vi "GEOM_GeomMngr.vi"(5 "calc headers?":bool=TRUE, 6 "arguments":string[](array[string]), 7 "hdrmodspath":path=path "kk", 8 "error in (no error)":errorcluster, 9 "switches":string[](array[string]), 10 "command":string, 11 "database path":path=path "/home/ArcVIEW/Modules/GEOM/public/database") -> (0 "error out":errorcluster, 2 "response":string)   [LabVIEW 2016]
uses:
  GEOM_Coords.ctl
  GEOM_FPAReadMode.ctl
  GEOM_Amplifier.ctl
  GEOM_AmpType.ctl
  GEOM_ROI.ctl
  GEOM_ROICorrection.ctl
  GEOM_CoordsRef.ctl
  GEOM_VAR_action.ctl
  GEOM_Gbls.vi
panel:
  out "ref":T1
  in  "GEOM_coordsref":T1
  out "lastformat":string
  in  "BinCorrectionType":T2(ring)
  out "last readmode":string
  in  "CorrectionType":T3
  in  "FPAReadMode":T4 {"Amplifiers"."fliped" items=["none", "horizontal", "vertical"]; "Amplifiers"."type" items=["LL", "LR", "UL", "UR"]}
  in  "ROIcoords":T8={"xstart"=1, "ystart"=1, "xsize"=1, "ysize"=1}
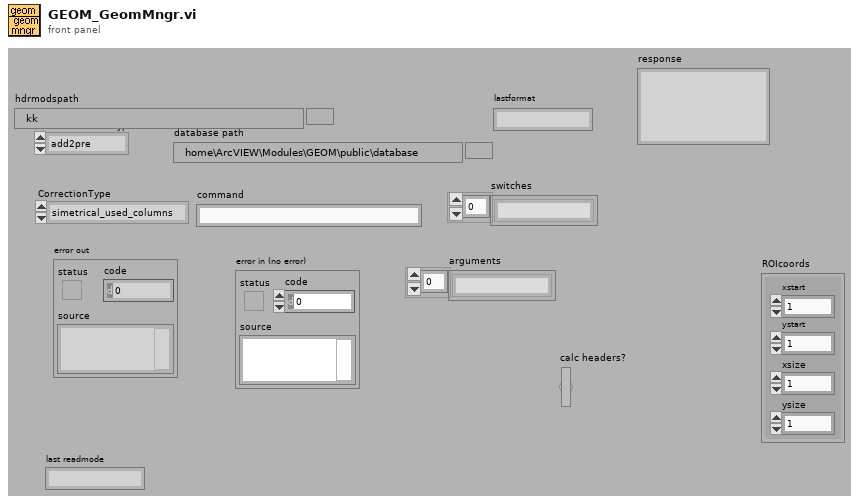
[diagram p1: front panel]
types:
  T1 = typedef "GEOM_CoordsRef.ctl" = cluster{"xref":u32, "yref":u32}
  T2 = enum16{"add2pre", "add2post", "add2data", "none"}
  T3 = typedef "GEOM_ROICorrection.ctl" = enum16{"simetrical_used_columns", "simetrical_all_columns"}
  T4 = typedef "GEOM_FPAReadMode.ctl" = cluster{"name":string, "Amplifiers":T5[]}
  T5 = typedef "GEOM_Amplifier.ctl" = cluster{"number":i32, "type":T6, "rotated":i16, "fliped":u16, "FPAcoord":cluster{"xstart":i32, "ystart":i32}, "Physical_size":cluster{"columns":i32, "rows":i32}, "predata":cluster{"columns":i32, "rows":i32}, "postdata":cluster{"columns":i32, "rows":i32}, "Req ROIs":T7, "Corr ROI":T7, "Detnumber":i32, "ampID":string, "discard":i32}
  T6 = typedef "GEOM_AmpType.ctl" = u16
  T7 = typedef "GEOM_ROI.ctl" = T8[]
  T8 = typedef "GEOM_Coords.ctl" = cluster{"xstart":u32, "ystart":u32, "xsize":u32, "ysize":u32}
  T9 = typedef "GEOM_VAR_action.ctl" = enum16{"read", "write"}
  T10 = typedef "DatabaseHand_RefNum.ctl" = refnum<vi>
  T11 = typedef "GEOM_AmpModifiers.ctl" = cluster{"Binning":T12, "sections":T13[]}
  T12 = typedef "GEOM_Binning.ctl" = cluster{"x":u32, "y":u32}
  T13 = typedef "GEOM_Moifier.ctl" = cluster{"name":string, "header section":string, "comment":string, "value":i32, "binning?":bool, "Where":enum16{"predata", "postdata"}, "add In":enum16{"columns", "rows", "none"}}
  T14 = typedef "GEOM_FPADetectors.ctl" = T15[]
  T15 = typedef "GEOM_DetStruct.ctl" = cluster{"name":string, "number":i32, "Info":string[][], "ReadModes":T16[], "detxpos":i32, "detypos":i32, "detcols":i32, "detrows":i32, "discard":i32}
  T16 = typedef "GEOM_ReadMode.ctl" = cluster{"name":string, "amplifiers":T5[], "nxamps":i32, "nyamps":i32}
  T17 = cluster{"FPA":string, "Info":string[][], "Sorted Detectors":T14}
  T18 = typedef "GEOM_DetSummaryStruct.ctl" = cluster{"detxpos":i32, "detypos":i32, "cols":i32, "rows":i32, "nxamps":i32, "nyamps":i32, "number":i32, "discard":i32, "totcols":i32, "totrows":i32, "readmode":string}
  T19 = typedef "GEOM_CorrectedFPA.ctl" = cluster{"readmode":string, "amplifiers":cluster{"number":i32, "xstart":i32, "ystart":i32}[], "totxsize":i32, "totysize":i32, "maxxdim":i32, "maxydim":i32, "numxamps":i32, "numyamps":i32, "totxdata":i32, "totydata":i32, "xdataamp":i32, "ydataamp":i32, "totpixels":i32}
  T20 = cluster{"name":string, "header section":string, "comment":string, "value":i32, "binning?":bool, "Where":enum16{"predata", "postdata"}, "add In":enum16{"columns", "rows", "none"}}[]
  T21 = cluster{"Amplifiers":T5[], "BinFPA":T19, "detreadmode":cluster{"name":string, "detectors":T18[]}}
  T22 = typedef "GEOM_HeaderModule.ctl" = cluster{"name":string, "Keys":string[][]}
  T23 = typedef "GEOM_HdrSec.ctl" = cluster{"name":string, "directives":T24, "comment":string, "amptype":enum16{"LL", "LR", "UL", "UR", "ALL", "LEFT", "RIGHT", "UPPER", "LOWER"}, "ampid":bool, "detid":bool, "unbin":bool}
  T24 = typedef "GEOM_CoorSys.ctl" = cluster{"coords":string, "reference":string, "xarea":string, "yarea":string, "order":string}
  T25 = typedef "GEOM_FormatGeomkeys.ctl" = cluster{"inienclose":string, "endenclose":string, "rangesep":string, "secsep":string}
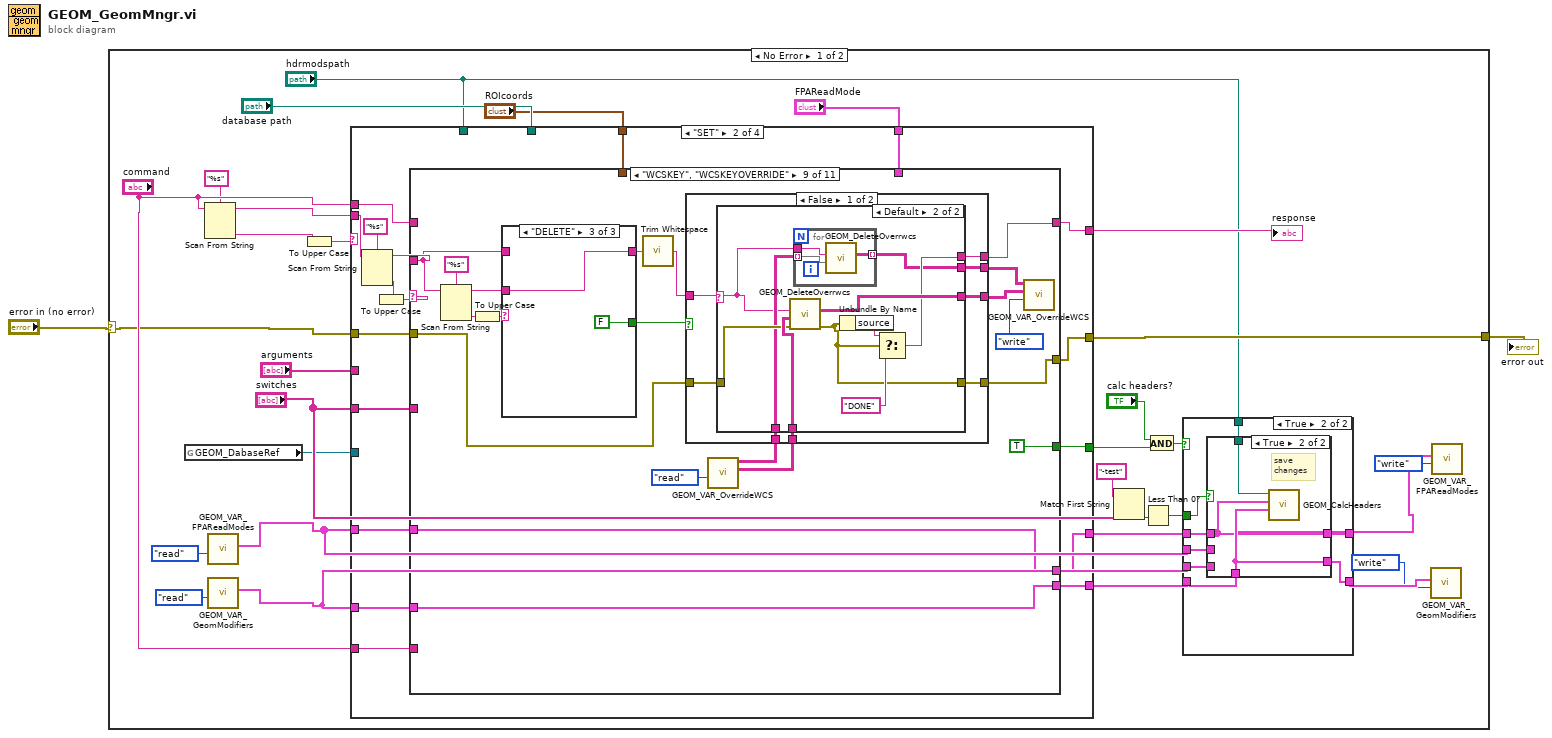
[diagram p0: block diagram]
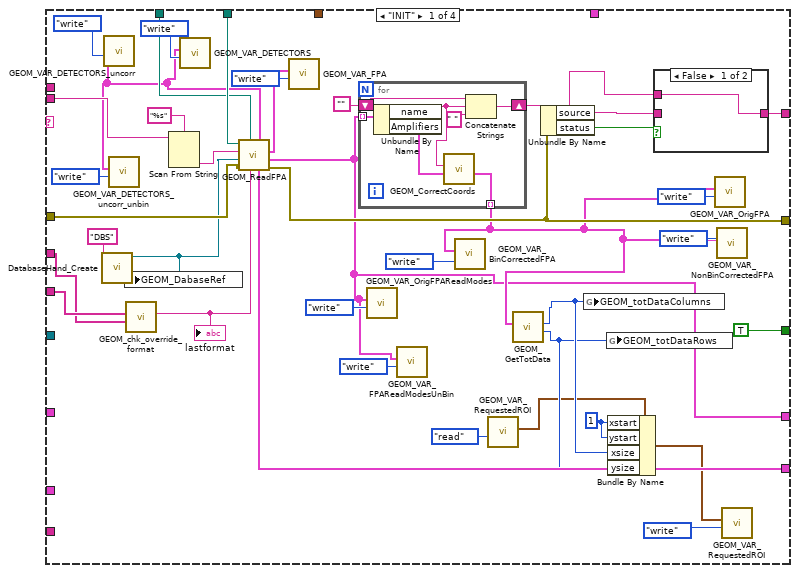
[diagram p2: hidden frame]
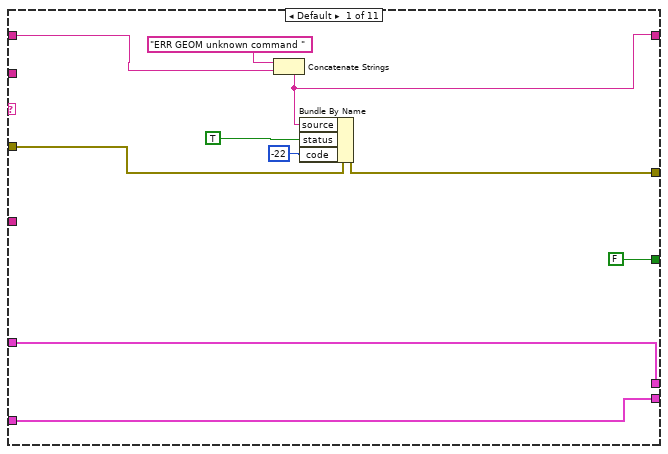
[diagram p4: hidden frame]
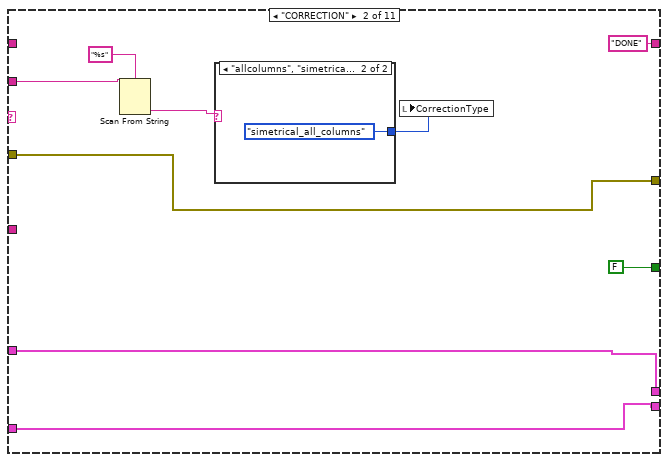
[diagram p5: hidden frame]
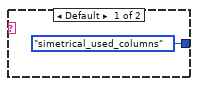
[diagram p6: hidden frame]
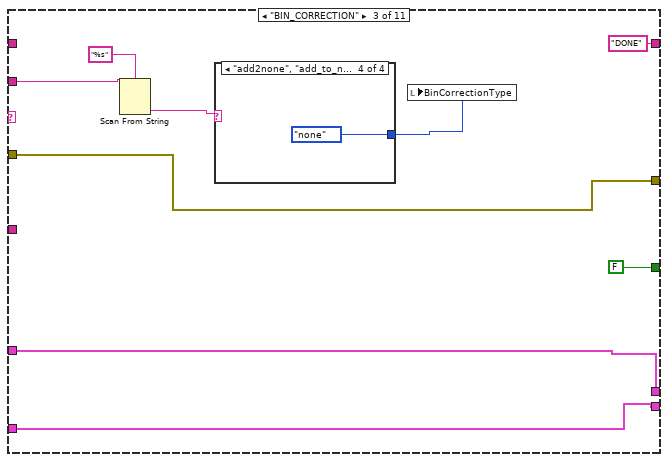
[diagram p7: hidden frame]
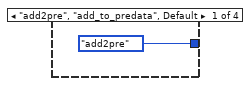
[diagram p8: hidden frame]
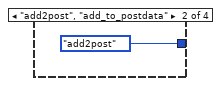
[diagram p9: hidden frame]
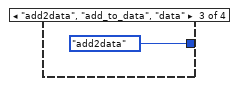
[diagram p10: hidden frame]
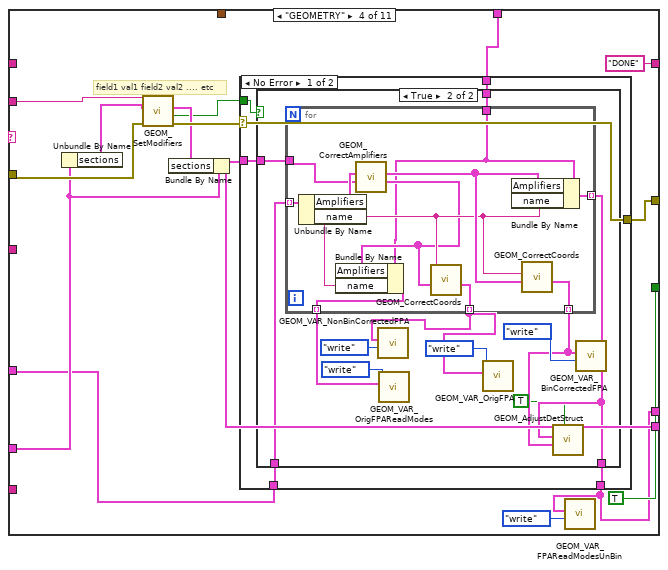
[diagram p11: hidden frame]
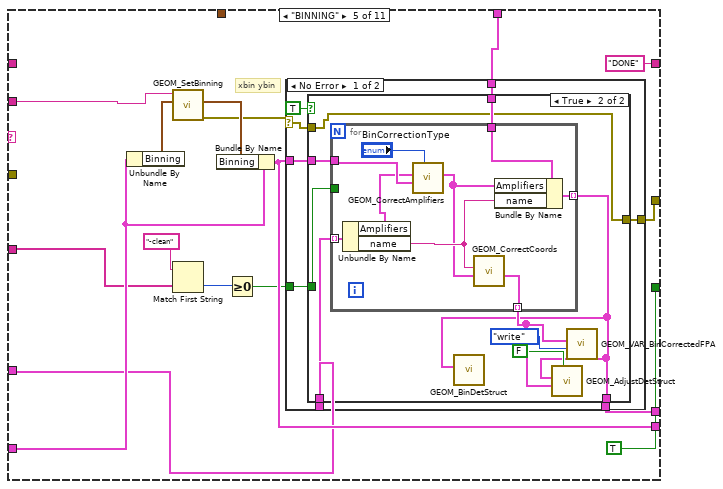
[diagram p14: hidden frame]
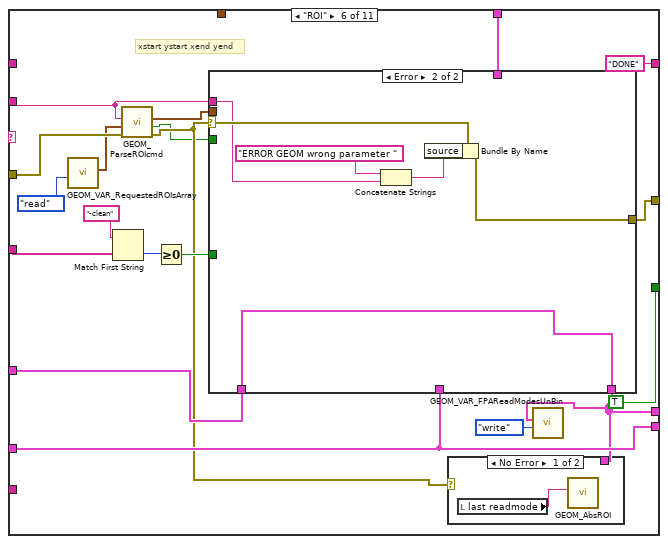
[diagram p17: hidden frame]
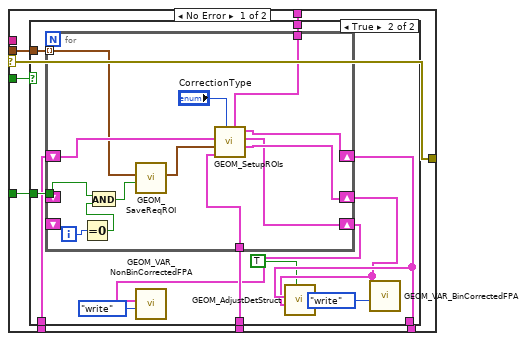
[diagram p19: hidden frame]
diagram:
  n1 = case shown="No Error" "error in (no error)" {
    selector: "error in (no error)" -> [w19 w727]
    tunnel: [w20 w727] -> w2
    frame No Error {
      n2 = global read "GEOM_Gbls.vi" "GEOM_DabaseRef"() -> (w18:T10)
      n3 = Scan From String(format string="%s", input string="command") -> (remaining string=w25:string, output 1=w26:string)  [unwired: 2 in, 3 out]
      n4 = call "GEOM_VAR_FPAReadModes.vi"("Action"=GEOM_VAR_action."read") -> ("GEOM_FPAReadModes out"=w14:T4[])  [unwired: 1 in, 9 out]
      n5 = call "GEOM_VAR_GeomModifiers.vi"("Action"=GEOM_VAR_action."read") -> ("GEOM_modifiers out"=w10:T11)  [unwired: 1 in, 9 out]
      n6 = To Upper Case(1:w26) -> (0:w7:string)
      n7 = case shown="\"SET\"" w7 {
        tunnel: "database path" -> [w72 _ _ _]
        tunnel: w19 -> [w39 w97 w409 w709]
        tunnel: [w67 w96 w408 w708] -> w20
        tunnel: w25 -> [w69 w95 w406 _]
        tunnel: "command" -> [_ w94 _ w706]
        tunnel: "switches" -> [w56 w86 _ _]
        tunnel: "ROIcoords" -> [_ w92 _ _]
        tunnel: "FPAReadMode" -> [_ w91 _ _]
        tunnel: w14 -> [_ w90 w410 w710]
        tunnel: [w34 w89 w410 w710] -> w22
        tunnel: w10 -> [_ w88 w407 w707]
        tunnel: [w68 w87 w407 w707] -> w21
        tunnel: [w65 w85 w411 w711] -> w29
        tunnel: "command" -> [_ w84 _ _]
        tunnel: w18 -> [_ _ w404 _]
        tunnel: "arguments" -> [w55 _ _ _]
        tunnel: "hdrmodspath" -> [w44 _ w400 _]
        tunnel: [TRUE ("x") w82 w401 FALSE ("x")] -> w6
        frame "INIT" {
          w60 = u32 1 ("xstart")
          n8 = call "DatabaseHand_Create.vi"("Name"="DBS") -> ("Database RefNum out"=w38:T10)  [unwired: 1 in, 9 out]
          n9 = global write "GEOM_Gbls.vi" "GEOM_DabaseRef"(w38) -> ()
          n10 = call "GEOM_chk_override_format.vi"("arguments"=w55, "switches"=w56) -> ("format out"=w57:string)  [unwired: 9 out]
          "lastformat" <- w57
          n11 = Scan From String(format string="%s", input string=w69) -> (output 1=w70:string)  [unwired: 2 in, 4 out]
          n12 = call "GEOM_ReadFPA.vi"("override format"=w57, "moddir"=w44, "error in (no error)"=w39, "Database RefNum out"=w38, "FPA"=w70, "database path"=w72) -> ("error out"=w67:errorcluster, "FPAReadModes"=w34:T4[], "FPA"=w49:T17, "modifiers"=w68:T11, "detreadmodes"=w36:cluster{"name":string, "detectors":T18[]}[])  [unwired: 1 out]
          n13 = call "GEOM_VAR_DETECTORS_uncorr.vi"("Action"=GEOM_VAR_action."write", "det in"=w36) -> ()  [unwired: 10 out]
          n14 = call "GEOM_VAR_DETECTORS_uncorr_unbin.vi"("Action"=GEOM_VAR_action."write", "det in"=w36) -> ()  [unwired: 10 out]
          n15 = call "GEOM_VAR_DETECTORS.vi"("Action"=GEOM_VAR_action."write", "det in"=w36) -> ()  [unwired: 10 out]
          n16 = call "GEOM_VAR_FPA.vi"("Action"=GEOM_VAR_action."write", "GEOM_FPA"=w49) -> ()  [unwired: 10 out]
          n17 = for {
            tunnel: w34 -> [w79] mode=indexing
            shift-right: [w77] -> w62
            shift-left: "" -> [w78]
            tunnel: [w73] -> w52 mode=indexing
            n18 = Unbundle By Name(w79) -> ("name"=w74:string, "Amplifiers"=w75:T5[])
            n19 = call "GEOM_CorrectCoords.vi"("Amplifiers"=w75, "readmode"=w74) -> ("correctedReadMode"=w73:T19)  [unwired: 9 out]
            n20 = Concatenate Strings(w78, w74, " " ("string")) -> (w77:string)
          }
          n21 = call "GEOM_VAR_OrigFPAReadModes.vi"("Action"=GEOM_VAR_action."write", "GEOM_OrigFPAReadModes"=w34) -> ()  [unwired: 10 out]
          n22 = call "GEOM_VAR_FPAReadModesUnBin.vi"("Action"=GEOM_VAR_action."write", "GEOM_FPAReadModes"=w34) -> ()  [unwired: 10 out]
          n23 = call "GEOM_VAR_BinCorrectedFPA.vi"("Action"=GEOM_VAR_action."write", "GEOM_BinCorrectedFPA in"=w52) -> ()  [unwired: 10 out]
          n24 = call "GEOM_VAR_RequestedROI.vi"("Action"=GEOM_VAR_action."read") -> ("GEOM_RequestedROI out"=w46:T8)  [unwired: 1 in, 9 out]
          n25 = call "GEOM_GetTotData.vi"("CorrectedFPA"=w52) -> ("tot data rows"=w58:i32, "tot data columns"=w59:i32)  [unwired: 9 out]
          n26 = Unbundle By Name(w67) -> ("source"=w64:string, "status"=w66:bool)
          n27 = global write "GEOM_Gbls.vi" "GEOM_totDataColumns"(w59) -> ()
          n28 = global write "GEOM_Gbls.vi" "GEOM_totDataRows"(w58) -> ()
          n29 = Bundle By Name(cluster=w46, "xstart"=w60, "ystart"=w60, "xsize"=w59, "ysize"=w58) -> (w43:T8)
          n30 = case shown="False" w66 {
            tunnel: w64 -> [_ w81]
            tunnel: [w80 w81] -> w65
            tunnel: w62 -> [w80 _]
            frame False {
            }
            frame True {
            }
          }
          n31 = call "GEOM_VAR_OrigFPA.vi"("Action"=GEOM_VAR_action."write", "GEOM_OrigFPA"=w52) -> ()  [unwired: 10 out]
          n32 = call "GEOM_VAR_NonBinCorrectedFPA.vi"("Action"=GEOM_VAR_action."write", "GEOM_NonBinCorrectedFPA in"=w52) -> ()  [unwired: 10 out]
          n33 = call "GEOM_VAR_RequestedROI.vi"("Action"=GEOM_VAR_action."write", "GEOM_RequestedROI"=w43) -> ()  [unwired: 10 out]
        }
        frame "SET" {
          n34 = Scan From String(format string="%s", input string=w95) -> (remaining string=w93:string, output 1=w98:string)  [unwired: 2 in, 3 out]
          n35 = To Upper Case(1:w98) -> (0:w83:string)
          n36 = case shown="\"WCSKEY\", \"WCSKEYOVERRIDE\"" w83 {
            tunnel: w97 -> [w106 w114 w126 w146 _ w236 w297 w311 w333 w391 w396]
            tunnel: [w105 w114 w126 w147 w194 w240 w297 w310 w332 w391 w396] -> w96
            tunnel: w94 -> [w104 _ _ _ _ _ _ _ _ _ _]
            tunnel: w86 -> [_ _ _ _ w185 w245 _ _ _ _ _]
            tunnel: w93 -> [_ w118 w129 w144 w193 w227 w296 w316 w343 w390 _]
            tunnel: w92 -> [_ _ _ _ _ _ _ _ _ _ _]
            tunnel: w91 -> [_ _ _ w148 w196 w241 _ _ _ _ _]
            tunnel: w90 -> [w103 w113 w125 w139 w182 w237 w290 w318 w350 w393 w398]
            tunnel: [w103 w113 w125 w134 w195 w228 w290 w318 w350 w393 w398] -> w89
            tunnel: w88 -> [w102 w112 w124 w142 w190 w239 w298 w317 w349 w394 w399]
            tunnel: [w102 w112 w124 w140 w188 w239 w298 w317 w349 w394 w399] -> w87
            tunnel: [w101 "DONE" ("source") "DONE" ("source") "DONE" ("source") "DONE" ("source") "DONE" ("source") w286 w309 w334 w389 "DONE" ("response")] -> w85
            tunnel: w84 -> [_ _ _ _ _ _ _ _ _ _ _]
            tunnel: [FALSE ("x") FALSE ("x") FALSE ("x") TRUE ("x") TRUE ("x") TRUE ("x") TRUE ("x") TRUE ("x") TRUE ("x") TRUE ("x") TRUE ("x")] -> w82
            frame Default {
              n37 = Concatenate Strings("ERR GEOM unknown command " ("source"), w104) -> (w101:string)
              n38 = Bundle By Name(cluster=w106, "source"=w101, "status"=TRUE, "code"=-22) -> (w105:errorcluster)
            }
            frame "CORRECTION" {
              n39 = Scan From String(format string="%s", input string=w118) -> (output 1=w116:string)  [unwired: 2 in, 4 out]
              n40 = case shown="\"allcolumns\", \"simetrical_all_columns\"" w116 {
                tunnel: [GEOM_ROICorrection."simetrical_used_columns" ("CorrectionType") GEOM_ROICorrection."simetrical_all_columns" ("CorrectionType")] -> w115
                frame Default {
                }
                frame "allcolumns", "simetrical_all_columns" {
                }
              }
              n41 = local write "CorrectionType"(w115) -> ()
            }
            frame "BIN_CORRECTION" {
              n42 = Scan From String(format string="%s", input string=w129) -> (output 1=w127:string)  [unwired: 2 in, 4 out]
              n43 = case shown="\"add2none\", \"add_to_none\", \"discard\", \"none\"" w127 {
                tunnel: [T2."add2pre" ("BinCorrectionType") T2."add2post" ("BinCorrectionType") T2."add2data" ("BinCorrectionType") T2."none" ("BinCorrectionType")] -> w122
                frame "add2pre", "add_to_predata", Default {
                }
                frame "add2post", "add_to_postdata" {
                }
                frame "add2data", "add_to_data", "data" {
                }
                frame "add2none", "add_to_none", "discard", "none" {
                }
              }
              n44 = local write "BinCorrectionType"(w122) -> ()
            }
            frame "GEOMETRY" {
              # "field1 val1 field2 val2 .... etc"
              n45 = Unbundle By Name(w142) -> ("sections"=w143:T13[])
              n46 = call "GEOM_SetModifiers.vi"("error in (no error)"=w146, "sections in"=w143, "sections string"=w144) -> ("error out"=w145:errorcluster, "changed"=w137:bool, "sections out"=w141:T20)  [unwired: 6 out]
              n47 = Bundle By Name(cluster=w142, "sections"=w141) -> (w140:T11)
              n48 = case shown="No Error" w145 {
                selector: w145 -> [w154 w179]
                tunnel: [w154 w179] -> w147
                tunnel: w148 -> [w153 _]
                tunnel: w139 -> [w152 w180]
                tunnel: [w150 w180] -> w134
                tunnel: w140 -> [w151 _]
                tunnel: w137 -> [w149 _]
                frame No Error {
                  n49 = case shown="True" w149 {
                    tunnel: w153 -> [_ w167]
                    tunnel: w152 -> [w155 w166]
                    tunnel: w151 -> [_ w165]
                    tunnel: [w155 w158] -> w150
                    frame False {
                    }
                    frame True {
                      n50 = for {
                        tunnel: w166 -> [w170] mode=indexing
                        tunnel: [w178] -> w158 mode=indexing
                        tunnel: w167 -> [w169]
                        tunnel: w165 -> [w176]
                        tunnel: [w174] -> w157 mode=indexing
                        tunnel: [w172] -> w162 mode=indexing
                        tunnel: [w168] -> w160 mode=indexing
                        n51 = Unbundle By Name(w170) -> ("Amplifiers"=w177:T5[], "name"=w173:string)
                        n52 = call "GEOM_CorrectAmplifiers.vi"("modifiers"=w176, "Amplifiers"=w177) -> ("NonBinnedAmplifiers"=w171:T5[], "BinnedAmplifiers"=w175:T5[])  [unwired: 2 in, 6 out]
                        n53 = Bundle By Name(cluster=w169, "Amplifiers"=w171, "name"=w173) -> (w168:T4)
                        n54 = call "GEOM_CorrectCoords.vi"("Amplifiers"=w171, "readmode"=w173) -> ("correctedReadMode"=w172:T19)  [unwired: 9 out]
                        n55 = Bundle By Name(cluster=w169, "Amplifiers"=w175, "name"=w173) -> (w178:T4)
                        n56 = call "GEOM_CorrectCoords.vi"("Amplifiers"=w175, "readmode"=w173) -> ("correctedReadMode"=w174:T19)  [unwired: 9 out]
                      }
                      n57 = call "GEOM_VAR_NonBinCorrectedFPA.vi"("Action"=GEOM_VAR_action."write", "GEOM_NonBinCorrectedFPA in"=w162) -> ()  [unwired: 10 out]
                      n58 = call "GEOM_VAR_OrigFPAReadModes.vi"("Action"=GEOM_VAR_action."write", "GEOM_OrigFPAReadModes"=w160) -> ()  [unwired: 10 out]
                      n59 = call "GEOM_VAR_OrigFPA.vi"("Action"=GEOM_VAR_action."write", "GEOM_OrigFPA"=w162) -> ()  [unwired: 10 out]
                      n60 = call "GEOM_AdjustDetStruct.vi"("corr unbin"=TRUE ("corr uncorr"), "GEOM_CorrectedFPA in"=w157, "GEOM_FPAReadModes"=w158) -> ()  [unwired: 9 out]
                      n61 = call "GEOM_VAR_BinCorrectedFPA.vi"("Action"=GEOM_VAR_action."write", "GEOM_BinCorrectedFPA in"=w157) -> ()  [unwired: 10 out]
                    }
                  }
                }
                frame Error {
                }
              }
              n62 = call "GEOM_VAR_FPAReadModesUnBin.vi"("Action"=GEOM_VAR_action."write", "GEOM_FPAReadModes"=w134) -> ()  [unwired: 10 out]
            }
            frame "BINNING" {
              # "xbin ybin"
              n63 = Unbundle By Name(w190) -> ("Binning"=w192:T12)
              n64 = call "GEOM_SetBinning.vi"("Binning In"=w192, "binning string"=w193) -> ("error out"=w189:errorcluster, "Binning Out"=w191:cluster{"x":u32, "y":u32})  [unwired: 1 in, 7 out]
              n65 = Match First String(2:w185, 3:"-clean" ("string")) -> (0:w186:i32)  [unwired: 1 out]
              n66 = Bundle By Name(cluster=w190, "Binning"=w191) -> (w188:T11)
              n67 = Greater Or Equal To 0?(x=w186) -> (x >= 0?=w184:bool)
              n68 = case shown="No Error" w189 {
                selector: w189 -> [w199 w225]
                tunnel: [w198 w225] -> w194
                tunnel: w196 -> [w204 _]
                tunnel: w182 -> [w203 w226]
                tunnel: [w202 w226] -> w195
                tunnel: w188 -> [w201 _]
                tunnel: w184 -> [w200 _]
                frame No Error {
                  n69 = case shown="True" TRUE {
                    tunnel: w204 -> [_ w215]
                    tunnel: w203 -> [w206 w214]
                    tunnel: [w206 w207] -> w202
                    tunnel: w201 -> [_ w213]
                    tunnel: w200 -> [_ w212]
                    tunnel: w199 -> [w205 w210]
                    tunnel: [w205 w210] -> w198
                    frame False {
                    }
                    frame True {
                      n70 = for {
                        tunnel: w214 -> [w221] mode=indexing
                        tunnel: [w224] -> w207 mode=indexing
                        tunnel: w215 -> [w223]
                        tunnel: w213 -> [w222]
                        tunnel: w212 -> [_]
                        tunnel: [w219] -> w209 mode=indexing
                        n71 = Unbundle By Name(w221) -> ("Amplifiers"=w218:T5[], "name"=w220:string)
                        n72 = call "GEOM_CorrectAmplifiers.vi"("BinCorrectionType"="BinCorrectionType", "modifiers"=w222, "Amplifiers"=w218) -> ("BinnedAmplifiers"=w217:T5[])  [unwired: 1 in, 7 out]
                        n73 = call "GEOM_CorrectCoords.vi"("Amplifiers"=w217, "readmode"=w220) -> ("correctedReadMode"=w219:T19)  [unwired: 9 out]
                        n74 = Bundle By Name(cluster=w223, "Amplifiers"=w217, "name"=w220) -> (w224:T4)
                      }
                      n75 = call "GEOM_BinDetStruct.vi"("GEOM_FPAReadModes"=w207) -> ()  [unwired: 11 out]
                      n76 = call "GEOM_AdjustDetStruct.vi"("corr unbin"=FALSE ("corr uncorr"), "GEOM_CorrectedFPA in"=w209, "GEOM_FPAReadModes"=w207) -> ()  [unwired: 9 out]
                      n77 = call "GEOM_VAR_BinCorrectedFPA.vi"("Action"=GEOM_VAR_action."write", "GEOM_BinCorrectedFPA in"=w209) -> ()  [unwired: 10 out]
                    }
                  }
                }
                frame Error {
                }
              }
            }
            frame "ROI" {
              # "xstart ystart xend yend"
              n78 = call "GEOM_VAR_RequestedROIsArray.vi"("Action"=GEOM_VAR_action."read") -> ("ROIs out"=w232:T8[])  [unwired: 1 in, 9 out]
              n79 = Match First String(2:w245, 3:"-clean" ("string")) -> (0:w243:i32)  [unwired: 1 out]
              n80 = call "GEOM_ParseROIcmd.vi"("error in"=w236, "current rois"=w232, "cmd"=w227) -> ("error out"=w234:errorcluster, "changed"=w231:bool, "req rois"=w235:T8[])  [unwired: 6 out]
              n81 = Greater Or Equal To 0?(x=w243) -> (x >= 0?=w242:bool)
              n82 = case shown="Error" w234 {
                selector: w234 -> [w254 w285]
                tunnel: w242 -> [w251 _]
                tunnel: [w254 w282] -> w240
                tunnel: w241 -> [w253 _]
                tunnel: w237 -> [w250 w281]
                tunnel: [w247 w281] -> w228
                tunnel: w239 -> [w252 _]
                tunnel: w235 -> [w249 _]
                tunnel: w231 -> [w248 _]
                tunnel: w227 -> [_ w280]
                frame No Error {
                  n83 = case shown="True" w248 {
                    tunnel: w253 -> [_ w266]
                    tunnel: w252 -> [_ w265]
                    tunnel: w251 -> [_ w264]
                    tunnel: w250 -> [w255 w263]
                    tunnel: w249 -> [_ w262]
                    tunnel: [w255 w258] -> w247
                    frame False {
                    }
                    frame True {
                      n84 = for {
                        tunnel: w266 -> [w278]
                        tunnel: w265 -> [w277]
                        tunnel: w264 -> [w270]
                        shift-right: [w273] -> w258
                        shift-left: w263 -> [w275]
                        tunnel: w262 -> [w274] mode=indexing
                        shift-right: [w272] -> w257
                        shift-left: _ -> [_]
                        shift-right: [w271] -> w259
                        shift-left: _ -> [_]
                        i -> [w269]
                        n85 = Equal To 0?(x=w269) -> (x = 0?=w268:bool)
                        n86 = And(x=w270, y=w268) -> (x .and. y?=w267:bool)
                        n87 = call "GEOM_SaveReqROI.vi"("clean"=w267, "GEOM_RequestedROI"=w274) -> ("ROIs out"=w276:T8[])  [unwired: 9 out]
                        n88 = call "GEOM_SetupROIs.vi"("FPAReadMode"=w278, "CorrectionType"="CorrectionType", "GEOM_modifiers"=w277, "ROIs"=w276, "GEOM_FPAReadModes"=w275) -> ("bin corr fpa"=w272:T19[], "nbincorr fpa"=w271:T19[], "GEOM_FPAReadModes  out"=w273:T4[])  [unwired: 4 out]
                      }
                      n89 = call "GEOM_VAR_NonBinCorrectedFPA.vi"("Action"=GEOM_VAR_action."write", "GEOM_NonBinCorrectedFPA in"=w259) -> ()  [unwired: 10 out]
                      n90 = call "GEOM_AdjustDetStruct.vi"("corr unbin"=TRUE ("corr uncorr"), "GEOM_CorrectedFPA in"=w257, "GEOM_FPAReadModes"=w258) -> ()  [unwired: 9 out]
                      n91 = call "GEOM_VAR_BinCorrectedFPA.vi"("Action"=GEOM_VAR_action."write", "GEOM_BinCorrectedFPA in"=w257) -> ()  [unwired: 10 out]
                    }
                  }
                }
                frame Error {
                  n92 = Concatenate Strings("ERROR GEOM wrong parameter " ("source"), w280) -> (w283:string)
                  n93 = Bundle By Name(cluster=w285, "source"=w283) -> (w282:errorcluster)
                }
              }
              n94 = case shown="No Error" w234 {
                tunnel: w228 -> [_ _]
                frame No Error {
                  n95 = local read "last readmode"() -> (w246:string)
                  n96 = call "GEOM_AbsROI.vi"("readmode"=w246) -> ()  [unwired: 11 out]
                }
                frame Error {
                }
              }
              n97 = call "GEOM_VAR_FPAReadModesUnBin.vi"("Action"=GEOM_VAR_action."write", "GEOM_FPAReadModes"=w228) -> ()  [unwired: 10 out]
            }
            frame "EXTENSIONS" {
              n98 = Scan From String(format string="%s", input string=w296) -> (output 1=w294:string)  [unwired: 2 in, 4 out]
              n99 = To Upper Case(1:w294) -> (0:w293:string)
              n100 = Index Array(array=w290) -> (element=w291:T4)  [unwired: 1 in]
              n101 = Unbundle By Name(w291) -> ("Amplifiers"=w292:T5[])
              n102 = Array Size(array=w292) -> (size(s)=w289:i32)
              n103 = case shown="Default" w293 {
                tunnel: w296 -> [_ w304]
                tunnel: [w299 w302] -> w287
                tunnel: w289 -> [w300 _]
                frame "DEFAULT", "ORDERED" {
                  n104 = for {
                    N: w300 -> [_]
                    tunnel: [w301] -> w299 mode=indexing
                    i -> [w301]
                  }
                }
                frame Default {
                  n105 = call "CMN_Str2Arr.vi"("separator"="\\n", "string in"=w304) -> ("Array out"=w303:string[])  [unwired: 2 in, 7 out]
                  n106 = Decimal String To Number(string=w303) -> (number=w302:i32[])  [unwired: 3 out]
                }
              }
              n107 = call "GEOM_SetExtensionsOrder.vi"("extensions"=w287) -> ("response"=w286:string)  [unwired: 10 out]
            }
            frame "COORDSORIG", "OFFCOORDS", "ORIGCOORDS", "REFCOORDS" {
              n108 = Scan From String(format string="%d %d", input string=w316) -> (output 1=w308:i32, output 2=w307:i32)  [unwired: 2 in, 5 out]
              n109 = Less Or Equal To 0?(x=w308) -> (x <= 0?=w314:bool)
              n110 = Less Or Equal To 0?(x=w307) -> (x <= 0?=w313:bool)
              n111 = Or(x=w314, y=w313) -> (x .or. y?=w312:bool)
              n112 = case shown="False" w312 {
                tunnel: w311 -> [w320 w330]
                tunnel: [w320 w329] -> w310
                tunnel: ["DONE" ("format string") w326] -> w309
                tunnel: w308 -> [w322 _]
                tunnel: w307 -> [w321 _]
                frame False {
                  n113 = Bundle By Name(cluster="GEOM_coordsref", "xref"=w322, "yref"=w321) -> (w324:T1)
                  "ref" <- w324
                  n114 = call "GEOM_VAR_CoordsRef.vi"("Action"=GEOM_VAR_action."write", "GEOM_coordsref"=w324) -> ()  [unwired: 10 out]
                }
                frame True {
                  w326 = "ERROR corrds must be >0" ("format string")
                  n115 = Bundle By Name(cluster=w330, "status"=TRUE, "code"=-22, "source"=w326) -> (w329:errorcluster)
                }
              }
            }
            frame "WCSKEY", "WCSKEYOVERRIDE" {
              n116 = Scan From String(format string="%s", input string=w343) -> (remaining string=w345:string, output 1=w347:string)  [unwired: 2 in, 3 out]
              n117 = To Upper Case(1:w347) -> (0:w346:string)
              n118 = case shown="\"DELETE\"" w346 {
                tunnel: w345 -> [_ w385 w387]
                tunnel: [TRUE TRUE FALSE] -> w344
                tunnel: w343 -> [w383 _ _]
                tunnel: [w383 w385 w387] -> w341
                frame Default {
                }
                frame "ADD" {
                }
                frame "DELETE" {
                }
              }
              n119 = call <vilib>:"Trim Whitespace.vi"("string"=w341) -> ("trimmed string"=w340:string)  [unwired: 1 in]
              n120 = call "GEOM_VAR_OverrideWCS.vi"("Action"=GEOM_VAR_action."read") -> ("override headers out"=w338:string[][], "override mext"=w339:string[][][])  [unwired: 2 in, 7 out]
              n121 = case shown="False" w344 {
                tunnel: w340 -> [w351 w382]
                tunnel: w339 -> [w353 w377]
                tunnel: w338 -> [w358 w381]
                tunnel: [w357 w380] -> w336
                tunnel: [w352 w376] -> w335
                tunnel: [w356 "DONE" ("format string")] -> w334
                tunnel: w333 -> [w355 w378]
                tunnel: [w354 w378] -> w332
                frame False {
                  n122 = case shown="Default" w351 {
                    selector: w351 -> [_ w363]
                    tunnel: w358 -> [_ w372]
                    tunnel: [string[][] [] ("out") w371] -> w357
                    tunnel: ["DONE" ("t") w370] -> w356
                    tunnel: w355 -> [w359 w369]
                    tunnel: [w359 w367] -> w354
                    tunnel: w353 -> [_ w365]
                    tunnel: [string[][][] [] ("out") w364] -> w352
                    frame "_ALL_" {
                    }
                    frame Default {
                      n123 = call "GEOM_DeleteOverrwcs.vi"("error in (no error)"=w369, "curr arr"=w372, "extension data"=w363) -> ("error out"=w367:errorcluster, "out"=w371:string[][])  [unwired: 7 out]
                      n124 = for {
                        tunnel: w365 -> [w375] mode=indexing
                        tunnel: w363 -> [w374]
                        tunnel: [w373] -> w364 mode=indexing
                        n125 = call "GEOM_DeleteOverrwcs.vi"("curr arr"=w375, "extension data"=w374) -> ("out"=w373:string[][])  [unwired: 1 in, 8 out]
                      }
                      n126 = Unbundle By Name(w367) -> ("source"=w366:string)
                      n127 = Select(t=w366, s=w367, f="DONE" ("t")) -> (s? t:f=w370:string)
                    }
                  }
                }
                frame True {
                  n128 = call "GEOM_Line2Overrwcs.vi"("curr mult array"=w377, "curr arr"=w381, "extension data"=w382) -> ("mout"=w376:string[][][], "out"=w380:string[][])  [unwired: 7 out]
                }
              }
              n129 = call "GEOM_VAR_OverrideWCS.vi"("Action"=GEOM_VAR_action."write", "override headers"=w336, "override headers mext"=w335) -> ()  [unwired: 9 out]
            }
            frame "GEOMHDRMOD", "WCSMOD" {
              n130 = call "GEOM_SetWCSMod.vi"("args in"=w390) -> ("response"=w389:string)  [unwired: 10 out]
            }
            frame "RECALCHDRS" {
            }
          }
        }
        frame "GET" {
          n131 = call "GEOM_VAR_FPA.vi"("Action"=GEOM_VAR_action."read") -> ("GEOM_FPA out"=w403:T17)  [unwired: 1 in, 9 out]
          n132 = Scan From String(format string="%s", input string=w406) -> (remaining string=w405:string, output 1=w413:string)  [unwired: 2 in, 3 out]
          n133 = To Upper Case(1:w413) -> (0:w412:string)
          n134 = case shown="\"HDRMODS\", \"HEADER\", \"HEADERMODS\", \"HEADMODS\"" w412 {
            tunnel: w410 -> [_ _ w435 w463 _ _ w491 w507 _ _ _ _ _ _ _ _ _ _ w681]
            tunnel: [w416 w424 w439 w468 w482 w486 w496 w520 w539 w552 w563 w601 w608 w618 w624 w639 w667 w677 w680] -> w411
            tunnel: w409 -> [w422 w426 w438 w467 w483 w487 w495 w510 w538 w551 w566 w604 w614 w620 w627 w645 w674 w678 w687]
            tunnel: w406 -> [w419 _ _ _ _ _ _ _ _ _ _ _ _ _ _ _ _ _ _]
            tunnel: [w418 w426 w437 w466 w483 w487 w494 w519 w538 w551 w566 w604 w614 w620 w627 w645 w674 w678 w687] -> w408
            tunnel: w407 -> [_ _ _ _ _ _ _ w506 w537 _ _ _ _ _ _ _ _ _ _]
            tunnel: w405 -> [_ _ w436 w465 _ _ w493 w518 _ _ w567 _ _ _ _ w644 _ _ w684]
            tunnel: w403 -> [_ _ _ _ _ _ _ _ _ w547 w561 _ _ _ _ _ _ _ _]
            tunnel: w404 -> [_ _ w430 _ _ _ _ _ _ _ _ _ _ _ _ _ _ _ _]
            tunnel: [FALSE ("x") FALSE ("x") w427 FALSE ("x") FALSE ("x") FALSE ("x") FALSE ("x") FALSE ("x") FALSE ("x") FALSE ("x") FALSE ("x") FALSE ("x") FALSE ("x") FALSE ("x") FALSE ("x") FALSE ("x") FALSE ("x") FALSE ("x") FALSE ("x")] -> w401
            tunnel: w400 -> [_ _ _ _ _ _ _ w508 _ _ _ _ _ _ _ _ _ _ _]
            frame Default {
              n135 = Concatenate Strings("GEOM: unknown command " ("source"), w419) -> (w416:string)
              n136 = Bundle By Name(cluster=w422, "source"=w416, "status"=TRUE, "code"=-22) -> (w418:errorcluster)
            }
            frame "READMODES" {
              n137 = call "GEOM_GetReadModes.vi"() -> ("readmodes"=w425:string[])  [unwired: 11 out]
              n138 = call "CMN_Arr2Str.vi"("Array in"=w425) -> ("string out"=w424:string)  [unwired: 10 out]
            }
            frame "AMPLIFIERS" {
              # "readmode"
              n139 = Scan From String(format string="%s", input string=w436) -> (output 1=w429:string)  [unwired: 2 in, 4 out]
              n140 = call "GEOM_findReadMode.vi"("binning corrected?"=TRUE, "GEOM_FPAReadModes"=w435, "readmode"=w429) -> ("BinFPA"=w432:T19, "FPAReadMode"=w433:T4, "amp found"=w434:bool, "detreadmode"=w428:cluster{"name":string, "detectors":T18[]})  [unwired: 5 out]
              n141 = case shown="True" w434 {
                tunnel: w433 -> [_ w455]
                tunnel: [w446 w456] -> w439
                tunnel: w438 -> [w445 w454]
                tunnel: [w444 w454] -> w437
                tunnel: w432 -> [_ w451]
                tunnel: w430 -> [_ w453]
                tunnel: w429 -> [_ w452]
                tunnel: w428 -> [_ w448]
                tunnel: [FALSE ("x") FALSE ("x")] -> w427
                frame False {
                  w446 = "READMODE NOT FOUND" ("name")
                  n142 = Bundle By Name(cluster=w445, "source"=w446, "status"=TRUE, "code"=-22) -> (w444:errorcluster)
                }
                frame True {
                  n143 = Unbundle By Name(w455) -> ("Amplifiers"=w450:T5[])
                  n144 = Bundle("Amplifiers"=w450, "BinFPA"=w451, "detreadmode"=w448) -> (w449:T21)  [unwired: 1 out]
                  n145 = Flatten To String(anything=w449) -> (data string=w456:string)  [unwired: 1 in, 4 out]
                  n146 = call "GEOM_SetNampsxy.vi"("BinFPA"=w451, "Database RefNum in"=w453) -> ()  [unwired: 10 out]
                  n147 = call "GEOM_AbsROI.vi"("readmode"=w452) -> ()  [unwired: 11 out]
                  "last readmode" <- w452
                }
              }
            }
            frame "ORIGAMPLIFIERS" {
              # "readmode"
              n148 = Scan From String(format string="%s", input string=w465) -> (output 1=w464:string)  [unwired: 2 in, 4 out]
              n149 = call "GEOM_findReadMode.vi"("binning corrected?"=FALSE, "GEOM_FPAReadModes"=w463, "readmode"=w464) -> ("BinFPA"=w460:T19, "FPAReadMode"=w461:T4, "amp found"=w462:bool, "detreadmode"=w458:cluster{"name":string, "detectors":T18[]})  [unwired: 5 out]
              n150 = case shown="True" w462 {
                tunnel: w461 -> [_ w480]
                tunnel: [w474 w481] -> w468
                tunnel: w467 -> [w473 w479]
                tunnel: [w472 w479] -> w466
                tunnel: w460 -> [_ w477]
                tunnel: w458 -> [_ w475]
                frame False {
                  w474 = "READMODE NOT FOUND" ("name")
                  n151 = Bundle By Name(cluster=w473, "source"=w474, "status"=TRUE, "code"=-22) -> (w472:errorcluster)
                }
                frame True {
                  n152 = Unbundle By Name(w480) -> ("Amplifiers"=w478:T5[])
                  n153 = Bundle("Amplifiers"=w478, "BinFPA"=w477, "detreadmode"=w475) -> (w476:T21)  [unwired: 1 out]
                  n154 = Flatten To String(anything=w476) -> (data string=w481:string)  [unwired: 1 in, 4 out]
                }
              }
            }
            frame "ROI" {
              n155 = call "GEOM_GetRoi2Str.vi"() -> ("roi"=w482:string)  [unwired: 11 out]
            }
            frame "ROIS" {
              n156 = call "GEOM_ROIArr2Str.vi"() -> ("defined rois"=w486:string)  [unwired: 1 in, 10 out]
            }
            frame "SIZE" {
              # "readmode"
              n157 = Scan From String(format string="%s", input string=w493) -> (output 1=w492:string)  [unwired: 2 in, 4 out]
              n158 = call "GEOM_findReadMode.vi"("GEOM_FPAReadModes"=w491, "readmode"=w492) -> ("BinFPA"=w489:T19, "amp found"=w490:bool)  [unwired: 1 in, 7 out]
              n159 = case shown="True" w490 {
                tunnel: [w502 w505] -> w496
                tunnel: w495 -> [w501 w504]
                tunnel: [w500 w504] -> w494
                tunnel: w489 -> [_ w503]
                frame False {
                  w502 = "READMODE NOT FOUND" ("name")
                  n160 = Bundle By Name(cluster=w501, "source"=w502, "status"=TRUE, "code"=-22) -> (w500:errorcluster)
                }
                frame True {
                  n161 = Flatten To String(anything=w503) -> (data string=w505:string)  [unwired: 1 in, 4 out]
                }
              }
            }
            frame "HEADERS" {
              # "(type: MULT or SING)"
              # "readmode type"
              n162 = To Upper Case(1:w518) -> (0:w516:string)
              n163 = Scan From String(format string="%s %s", input string=w516) -> (output 1=w517:string, output 2=w514:string)  [unwired: 2 in, 5 out]
              n164 = call "GEOM_CalcHeaders.vi"("error in (no error)"=w510, "modifiers"=w506, "FPAReadModes"=w507, "moddir"=w508) -> ("error out"=w509:errorcluster)  [unwired: 7 out]
              n165 = call "GEOM_GetHeaders.vi"("error in (no error)"=w509, "readmode"=w517) -> ("error out"=w513:errorcluster, "S Headers"=w512:string[][], "ME Headers"=w515:string[][][])  [unwired: 1 in, 6 out]
              n166 = case shown="No Error" w513 {
                selector: w513 -> [w522 w531]
                tunnel: [w526 w535] -> w520
                tunnel: [w522 w534] -> w519
                tunnel: w515 -> [w525 _]
                tunnel: w514 -> [w524 _]
                tunnel: w512 -> [w523 _]
                frame No Error {
                  n167 = case shown="\"S\", \"SING\", \"SINGLE\"" w524 {
                    tunnel: [w528 w530] -> w526
                    tunnel: w525 -> [w527 _]
                    tunnel: w523 -> [_ w529]
                    frame Default {
                      n168 = Flatten To String(anything=w527) -> (data string=w528:string)  [unwired: 1 in, 4 out]
                    }
                    frame "S", "SING", "SINGLE" {
                      n169 = Flatten To String(anything=w529) -> (data string=w530:string)  [unwired: 1 in, 4 out]
                    }
                  }
                }
                frame Error {
                  w535 = "READMODE NOT FOUND" ("name")
                  n170 = Bundle By Name(cluster=w531, "source"=w535, "status"=TRUE, "code"=-22) -> (w534:errorcluster)
                }
              }
            }
            frame "MODIF", "MODIFIERS" {
              n171 = Flatten To String(anything=w537) -> (data string=w539:string)  [unwired: 1 in, 4 out]
            }
            frame "FPAINFO" {
              n172 = Unbundle By Name(w547) -> ("FPA"=w544:string, "Info"=w546:string[][], "Sorted Detectors"=w550:T14)
              n173 = for {
                tunnel: w550 -> [w558] mode=indexing
                tunnel: [w553] -> w549 mode=indexing
                n174 = Unbundle By Name(w558) -> ("name"=w555:string, "number"=w556:i32)
                n175 = Format Into String(format string="detector_%d = ", w556) -> (resulting string=w554:string)  [unwired: 2 in, 1 out]
                n176 = Build Array(w554, w555) -> (w553:string[])
              }
              n177 = Build Array("FPA" ("element"), w544) -> (w543:string[])
              n178 = Insert Into Array(array=w546, index (row)=0, new element=w543) -> (w541:string[][])  [unwired: 1 in]
              n179 = Insert Into Array(array=w541, new element=w549) -> (w548:string[][])  [unwired: 2 in]
              n180 = call "CMN_2DArr2Str.vi"("array in"=w548) -> ("string out"=w552:string)  [unwired: 1 in, 9 out]
            }
            frame "DETINFO" {
              n181 = Unbundle By Name(w561) -> ("Sorted Detectors"=w560:T14)
              n182 = Scan From String(format string="%d", input string=w567) -> (remaining string=w562:string, error out=w569:errorcluster, output 1=w568:i32)  [unwired: 2 in, 2 out]
              n183 = case shown="Error" w569 {
                tunnel: w567 -> [_ _]
                tunnel: w568 -> [w577 _]
                tunnel: [w576 w591] -> w564
                tunnel: w567 -> [_ w590]
                tunnel: [w575 w587] -> w565
                tunnel: w562 -> [_ _]
                tunnel: w560 -> [w574 w586]
                frame No Error {
                  n184 = while {
                    tunnel: w577 -> [w584]
                    tunnel: w574 -> [w585] mode=indexing
                    tunnel: [w579] -> w576
                    tunnel: [w578] -> w575
                    stop <- w580 stop-if-true
                    n185 = Unbundle By Name(w585) -> ("number"=w583:i32, "name"=w581:string, "Info"=w579:string[][])
                    n186 = Equal?(x=w584, y=w583) -> (x = y?=w582:bool)
                    n187 = Empty String/Path?(string/path=w581) -> (empty?=w578:bool)
                    n188 = Or(x=w582, y=w578) -> (x .or. y?=w580:bool)
                  }
                }
                frame Error {
                  n189 = Scan From String(format string="%s", input string=w590) -> (output 1=w588:string)  [unwired: 2 in, 4 out]
                  n190 = while {
                    tunnel: w586 -> [w598] mode=indexing
                    tunnel: [w596] -> w591
                    tunnel: w588 -> [w595]
                    tunnel: [w592] -> w587
                    stop <- w597 stop-if-true
                    n191 = Unbundle By Name(w598) -> ("name"=w594:string, "Info"=w596:string[][])  [unwired: 1 out]
                    n192 = Equal?(x=w595, y=w594) -> (x = y?=w593:bool)
                    n193 = Empty String/Path?(string/path=w594) -> (empty?=w592:bool)
                    n194 = Or(x=w593, y=w592) -> (x .or. y?=w597:bool)
                  }
                }
              }
              n195 = case shown="False" w565 {
                tunnel: w564 -> [w572 _]
                tunnel: [w571 "ERROR\ndetector not found" ("string out")] -> w563
                frame False {
                  n196 = call "CMN_2DArr2Str.vi"("array in"=w572) -> ("string out"=w571:string)  [unwired: 1 in, 9 out]
                }
                frame True {
                }
              }
            }
            frame "COORDSORIG", "OFFCOORDS", "ORIGCOORDS", "REFCOORDS" {
              n197 = call "GEOM_VAR_CoordsRef.vi"("Action"=GEOM_VAR_action."read") -> ("GEOM_coordsref out"=w605:T1)  [unwired: 1 in, 9 out]
              n198 = Unbundle By Name(w605) -> ("xref"=w603:u32, "yref"=w602:u32)
              n199 = Format Into String(format string="%d %d", w603, w602) -> (resulting string=w601:string)  [unwired: 2 in, 1 out]
            }
            frame "WCSKEY", "WCSKEYOVERRIDE", "WCSKEYS" {
              n200 = call "GEOM_VAR_OverrideWCS.vi"("Action"=GEOM_VAR_action."read") -> ("override headers out"=w613:string[][])  [unwired: 2 in, 8 out]
              n201 = call "CMN_2DArr2Str.vi"("separator"=" ", "array in"=w613) -> ("string out"=w609:string)  [unwired: 9 out]
              n202 = Empty String/Path?(string/path=w609) -> (empty?=w611:bool)
              n203 = Select(t="NONE", s=w611, f=w609) -> (s? t:f=w608:string)
            }
            frame "DETFORMAT", "LASTDETFORMAT" {
              n204 = property on="lastformat" class="Str"() -> ("Value"=w619:string)  [unwired: 2 in, 2 out]
              n205 = Empty String/Path?(string/path=w619) -> (empty?=w621:bool)
              n206 = Select(t="default", s=w621, f=w619) -> (s? t:f=w618:string)
            }
            frame "HDRMODS", "HEADER", "HEADERMODS", "HEADMODS" {
              n207 = call "GEOM_VAR_HeaderModules.vi"("Action"=GEOM_VAR_action."read") -> ("GEOM_HeaderModules out"=w625:T22[])  [unwired: 1 in, 9 out]
              n208 = for {
                tunnel: w625 -> [w636] mode=indexing
                shift-right: [w633] -> w624
                shift-left: "" -> [w632]
                n209 = Unbundle By Name(w636) -> ("name"=w631:string, "Keys"=w635:string[][])
                n210 = call "CMN_2DArr2Str.vi"("separator"=" / ", "array in"=w635) -> ("string out"=w634:string)  [unwired: 9 out]
                n211 = Concatenate Strings(w632, w631, ":" ("string"), "\n", w634) -> (w633:string)
              }
            }
            frame "GEOMDIRECTIVES", "WCSDIRECTIVES" {
              n212 = Scan From String(format string="%s", input string=w644) -> (output 1=w642:string)  [unwired: 2 in, 4 out]
              n213 = call "GEOM_VAR_CustomKeys.vi"("Action"=GEOM_VAR_action."read") -> ("dethdrs out"=w638:T23[], "shdrs out"=w637:T23[], "amphdrs out"=w640:T23[])  [unwired: 4 in, 4 out]
              n214 = To Lower Case(string=w642) -> (all lower case string=w641:string)
              n215 = case shown="\"ampext\", \"mef\"" w641 {
                tunnel: w640 -> [_ w654 _ _]
                tunnel: ["ERROR <ampext | detext | single>" w653 w658 w662] -> w639
                tunnel: w638 -> [_ _ w660 _]
                tunnel: w637 -> [_ _ _ w661]
                frame Default {
                }
                frame "ampext", "mef" {
                  w649 = "\n"
                  n216 = call "GEOM_GetWCSDirectives.vi"("hdrs"=w654) -> ("directives out"=w650:string)  [unwired: 10 out]
                  n217 = Concatenate Strings("[MEF]" ("string"), w649, "#multiple amplifier extensions" ("string"), w649, w650) -> (w653:string)
                }
                frame "detext", "medf" {
                  w655 = "\n"
                  n218 = call "GEOM_GetWCSDirectives.vi"("hdrs"=w660) -> ("directives out"=w656:string)  [unwired: 10 out]
                  n219 = Concatenate Strings("[MEDF]" ("string"), w655, "#multiple detector extensions" ("string"), w655, w656) -> (w658:string)
                }
                frame "sef", "single" {
                  w664 = "\n"
                  n220 = call "GEOM_GetWCSDirectives.vi"("hdrs"=w661) -> ("directives out"=w663:string)  [unwired: 10 out]
                  n221 = Concatenate Strings("[SEF]" ("string"), w664, "#single" ("string"), w664, w663) -> (w662:string)
                }
              }
            }
            frame "GEOMFORMAT", "WCSFORMAT" {
              n222 = call "GEOM_VAR_CustomKeys.vi"("Action"=GEOM_VAR_action."read") -> ("format out"=w673:T25)  [unwired: 4 in, 6 out]
              n223 = Unbundle By Name(w673) -> ("inienclose"=w671:string, "endenclose"=w670:string, "rangesep"=w669:string, "secsep"=w668:string)
              n224 = Format Into String(format string="enclose=%s %s\\nrangesep=%s\\naxesep=%s", w671, w670, w669, w668) -> (resulting string=w667:string)  [unwired: 2 in, 1 out]
            }
            frame "GEOMHDRMOD", "WCSMOD" {
              n225 = call "GEOM_GetWCSMod.vi"() -> ("response"=w677:string)  [unwired: 11 out]
            }
            frame "FPAGEOM", "FPATOPO", "GEOMINFO", "TOPOLOGY" {
              n226 = Scan From String(format string="%s", input string=w684) -> (error out=w683:errorcluster, output 1=w682:string)  [unwired: 2 in, 3 out]
              n227 = case shown="Error" w683 {
                tunnel: w682 -> [w690 _]
                tunnel: w681 -> [w689 w693]
                tunnel: [w688 w692] -> w680
                frame No Error {
                  n228 = call "GEOM_GetTopo_1readmode.vi"("GEOM_FPAReadModes"=w689, "readmode"=w690) -> ("strinfo"=w688:string)  [unwired: 9 out]
                }
                frame Error {
                  n229 = call "GEOM_VAR_BinCorrectedFPA.vi"("Action"=GEOM_VAR_action."read") -> ("GEOM_BinCorrectedFPA out"=w694:T19[])  [unwired: 1 in, 9 out]
                  n230 = for {
                    tunnel: w694 -> [w701] mode=indexing
                    tunnel: w693 -> [w699]
                    shift-right: [w698] -> w692
                    shift-left: "" -> [w696]
                    n231 = Unbundle By Name(w701) -> ("readmode"=w700:string)
                    n232 = call "GEOM_GetTopo_1readmode.vi"("GEOM_FPAReadModes"=w699, "readmode"=w700) -> ("strinfo"=w697:string)  [unwired: 9 out]
                    n233 = Concatenate Strings(w696, w697) -> (w698:string)
                  }
                }
              }
            }
          }
        }
        frame Default {
          n234 = Concatenate Strings("GEOM: unknown command " ("source"), w706) -> (w711:string)
          n235 = Bundle By Name(cluster=w709, "source"=w711, "status"=TRUE, "code"=-22) -> (w708:errorcluster)
        }
      }
      "response" <- w29
      n236 = Match First String(2:"switches", 3:"-test" ("string")) -> (0:w23:i32)  [unwired: 1 out]
      n237 = Less Than 0?(x=w23) -> (x < 0?=w3:bool)
      n238 = And(x="calc headers?", y=w6) -> (x .and. y?=w4:bool)
      n239 = case shown="True" w4 {
        tunnel: w22 -> [w712 w721]
        tunnel: w21 -> [w713 w719]
        tunnel: [w712 w714] -> w16
        tunnel: [w713 w716] -> w12
        tunnel: w14 -> [_ w715]
        tunnel: w10 -> [_ w717]
        tunnel: "hdrmodspath" -> [_ w720]
        tunnel: w3 -> [_ w718]
        frame False {
          # "do not recalc headers"
        }
        frame True {
          n240 = case shown="True" w718 {
            tunnel: w721 -> [_ w724]
            tunnel: w720 -> [_ w726]
            tunnel: w719 -> [_ w725]
            tunnel: w717 -> [w723 _]
            tunnel: [w723 w725] -> w716
            tunnel: w715 -> [w722 _]
            tunnel: [w722 w724] -> w714
            frame False {
              # "only\ntest, \ndo not\nsave"
            }
            frame True {
              # "save \nchanges"
              n241 = call "GEOM_CalcHeaders.vi"("modifiers"=w725, "FPAReadModes"=w724, "moddir"=w726) -> ()  [unwired: 1 in, 8 out]
            }
          }
        }
      }
      n242 = call "GEOM_VAR_GeomModifiers.vi"("Action"=GEOM_VAR_action."write", "GEOM_modifiers"=w12) -> ()  [unwired: 10 out]
      n243 = call "GEOM_VAR_FPAReadModes.vi"("Action"=GEOM_VAR_action."write", "GEOM_FPAReadModes"=w16) -> ()  [unwired: 10 out]
    }
    frame Error {
    }
  }
  "error out" <- w2
